vi "ConvertADCRegisters.vi"(11 "Registersx12x13x14":u8[](array[numeric]) format="%.0x") -> (3 "Data Out":i32)   [LabVIEW 2020, in "CTI-Peripheral.lvlib" / "Adafruit NAU7802 24bit Strain Gauge.lvclass"]
uses:
  Adafruit NAU7802 24bit Strain Gauge.lvclass
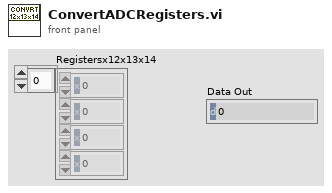
[diagram p1: front panel]
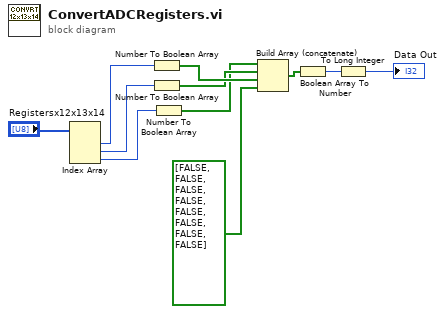
[diagram p0: block diagram]
diagram:
  n1 = Index Array(array="Registersx12x13x14") -> (element #1=w10:u8, element #2=w9:u8, element #3=w8:u8)  [unwired: 3 in]
  n2 = Number To Boolean Array(number=w10) -> (Boolean array=w7:bool[])
  n3 = Number To Boolean Array(number=w9) -> (Boolean array=w6:bool[])
  n4 = Number To Boolean Array(number=w8) -> (Boolean array=w5:bool[])
  n5 = Build Array (concatenate)(w5, w6, w7, bool[] [FALSE, FALSE, FALSE, FALSE, FALSE, FALSE, FALSE, FALSE] ("array")) -> (w4:bool[])
  n6 = Boolean Array To Number(Boolean array=w4) -> (number=w3:u32)
  n7 = To Long Integer(number=w3) -> (32bit integer=→"Data Out":i32)
